vi "RunTest_ReportsNotImplementedError.vi"() -> ()   [LabVIEW 2019, in "TestCaseTest.lvlib"]
uses:
  TestCaseTest.lvlib
  TestCase/TestCase/TestCase.lvclass
  Assertion/Assertion.lvlib
panel:
  out "error out":errorcluster
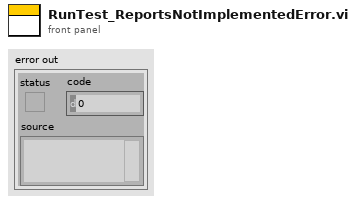
[diagram p1: front panel]
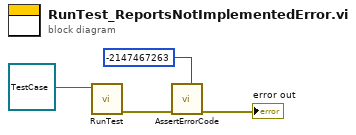
[diagram p0: block diagram]
diagram:
  n1 = call-dynamic "RunTest.vi"("TestCase in"=refnum<class "TestCase.lvclass"> refnum ("TestCase.lvlib:TestCase.lvclass")) -> ("error out"=w3:errorcluster)  [unwired: 9 in, 1 out]
  n2 = call "AssertErrorCode.vi"("Expected"=-2147467263, "error in (no error)"=w3) -> ("error out"=→"error out":errorcluster)  [unwired: 9 in]
